vi "Serial No.vi"(3 "Increment? (T)":bool=TRUE, 6 "Input S/N":string) -> (2 "Output S/N":string)   [LabVIEW 2011]
doc: "Searches backwards through a string to find the first continuous sub-string of integer numbers. This substring is converted to a number, incremented/decremented, and converted back to a substring. The original string is re-composed and output.\n\nDecrementing below 0 results in a 0. Incrementing above the available digits will add not add a digit (just cycle back to 0)."
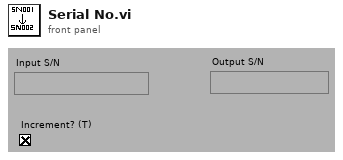
[diagram p1: front panel]
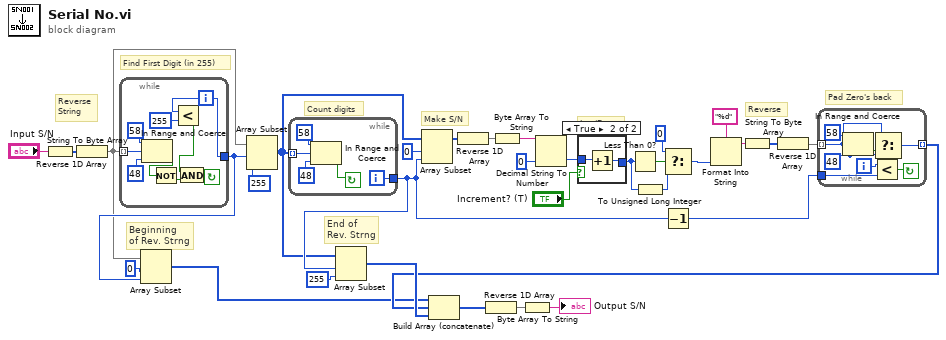
[diagram p0: block diagram]
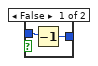
[diagram p2: hidden frame]
diagram:
  # "End of\nRev. Strng"
  # "Beginning\nof Rev. Strng"
  # "Reverse"
  # "Pad Zero's back"
  # "Incr/Decr"
  # "Make S/N"
  # "Reverse\nString"
  # "Count digits"
  # "Find First Digit (in 255)"
  n1 = String To Byte Array(string="Input S/N") -> (unsigned byte array=w6:u8[])
  n2 = Reverse 1D Array(array=w6) -> (reversed array=w22:u8[])
  n3 = while {
    tunnel: [w36] -> w25
    tunnel: w22 -> [w40] mode=indexing
    i -> [w36]
    stop <- w34 continue-if-true
    n4 = In Range and Coerce(upper limit=u8 58 ("hi"), x=w40, lower limit=u8 48 ("lo")) -> (In Range?=w37:bool)  [unwired: 1 out]
    n5 = Not(x=w37) -> (.not. x?=w41:bool)
    n6 = Less?(x=w36, y=255) -> (x < y?=w33:bool)
    n7 = And(x=w33, y=w41) -> (x .and. y?=w34:bool)
  }
  n8 = Array Subset(array=w22, index=0, length=w25) -> (w29:u8[])
  n9 = Array Subset(array=w22, index=w25, length=255) -> (w26:u8[])
  n10 = while {
    tunnel: [w43] -> w28
    tunnel: w26 -> [w46] mode=indexing
    i -> [w43]
    stop <- w42 continue-if-true
    n11 = In Range and Coerce(upper limit=u8 58 ("hi"), x=w46, lower limit=u8 48 ("lo")) -> (In Range?=w42:bool)  [unwired: 1 out]
  }
  n12 = Array Subset(array=w26, index=w28, length=255) -> (w32:u8[])
  n13 = Array Subset(array=w26, index=0, length=w28) -> (w10:u8[])
  n14 = Reverse 1D Array(array=w10) -> (reversed array=w11:u8[])
  n15 = Byte Array To String(unsigned byte array=w11) -> (string=w12:string)
  n16 = Decimal String To Number(string=w12, default (0L)=0) -> (number=w14:i32)  [unwired: 2 out]
  n17 = case shown="True" "Increment? (T)" {
    tunnel: w14 -> [w48 w50]
    tunnel: [w47 w49] -> w3
    frame False {
      n18 = Decrement(x=w48) -> (x-1=w47:i32)
    }
    frame True {
      n19 = Increment(x=w50) -> (x+1=w49:i32)
    }
  }
  n20 = Less Than 0?(x=w3) -> (x < 0?=w5:bool)
  n21 = To Unsigned Long Integer(number=w3) -> (unsigned 32bit integer=w1:u32)
  n22 = Select(t=u16 0, s=w5, f=w1) -> (s? t:f=w4:u32)
  n23 = Decrement(x=w28) -> (x-1=w20:i32)
  n24 = Format Into String(format string="%d", w4) -> (resulting string=w17:string)  [unwired: 2 in, 1 out]
  n25 = String To Byte Array(string=w17) -> (unsigned byte array=w18:u8[])
  n26 = Reverse 1D Array(array=w18) -> (reversed array=w19:u8[])
  n27 = while {
    tunnel: [w51] -> w31 mode=indexing
    tunnel: w20 -> [w56]
    tunnel: w19 -> [w53] mode=indexing
    i -> [w57]
    stop <- w55 continue-if-true
    w52 = u8 48 ("lo")
    n28 = In Range and Coerce(upper limit=u8 58 ("hi"), x=w53, lower limit=w52) -> (In Range?=w54:bool)  [unwired: 1 out]
    n29 = Less?(x=w57, y=w56) -> (x < y?=w55:bool)
    n30 = Select(t=w53, s=w54, f=w52) -> (s? t:f=w51:u8)
  }
  n31 = Build Array (concatenate)(w29, w31, w32) -> (w30:u8[])
  n32 = Reverse 1D Array(array=w30) -> (reversed array=w21:u8[])
  n33 = Byte Array To String(unsigned byte array=w21) -> (string=→"Output S/N":string)
